vi "main.vi"() -> (0 "error out":errorcluster)   [LabVIEW 2012]
uses:
  Global1.vi
  <vilib>/Utility/file.llb/Read From Spreadsheet File (string).vi
panel:
  out "element":string
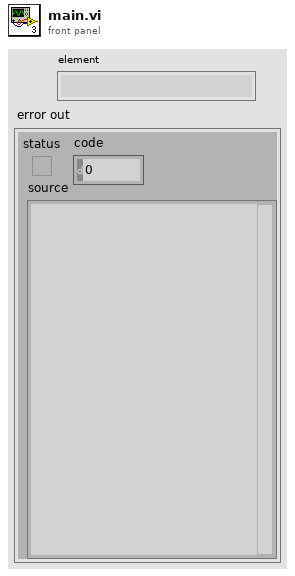
[diagram p1: front panel]
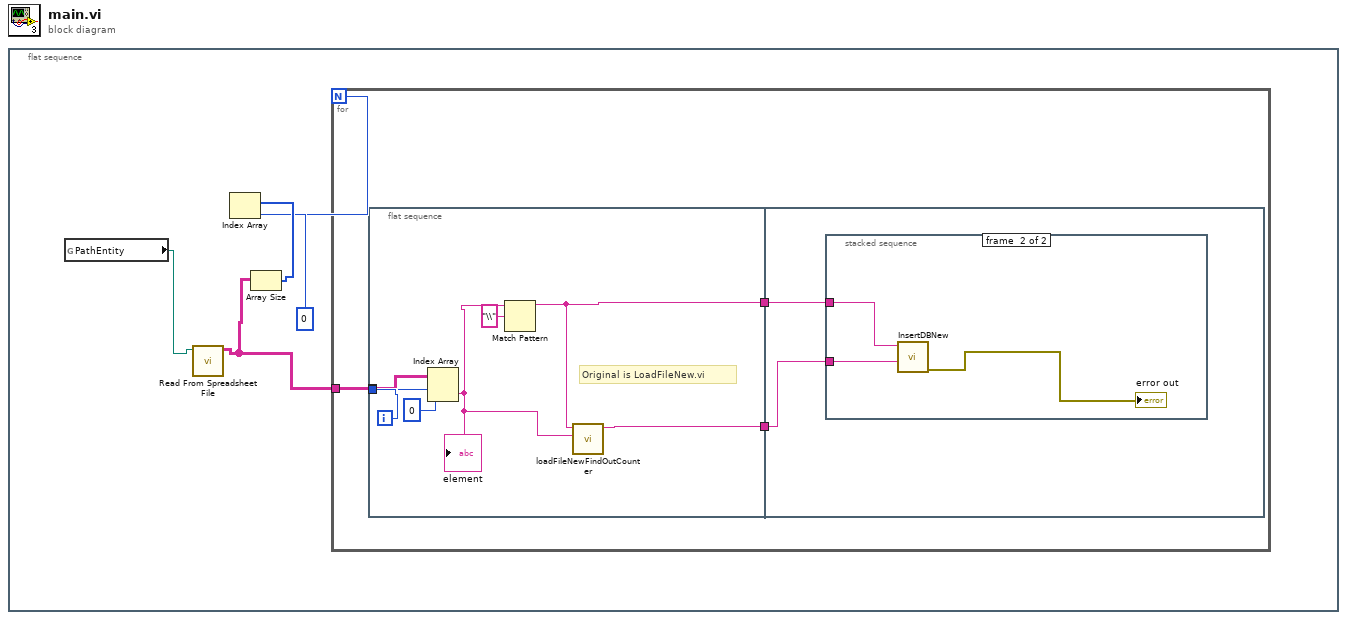
[diagram p0: block diagram]
diagram:
  n1 = flat-sequence {
    frame #0 {
      n2 = global read "Global1.vi" "PathEntity"() -> (w1:path)
      n3 = call-poly <vilib>:"Read From Spreadsheet File.vi"("file path (dialog if empty)"=w1) -> ("all rows"=w2:string[][])  [unwired: 6 in, 4 out]
      n4 = Array Size(array=w2) -> (size(s)=w5:i32[])
      n5 = Index Array(array=w5, index=0) -> (element=w3:i32)
      n6 = for {
        N: w3 -> [_]
        tunnel: w2 -> [w9]
        i -> [w8]
        n7 = flat-sequence {
          tunnel: w9 -> [w16]
          tunnel: w8 -> [w14]
          tunnel: [w11] -> w7
          tunnel: [w10] -> w6
          tunnel: w7 -> [w18]
          tunnel: w6 -> [w17]
          frame #0 {
            # "Original is LoadFileNew.vi"
            n8 = Index Array(array=w16, index (row)=w14, index (col)=0 ("disabled index (col)")) -> (element=w12:string)
            "element" <- w12
            n9 = Match Pattern(string=w12, regular expression="\\") -> (before substring=w10:string)  [unwired: 1 in, 3 out]
            n10 = call "loadFileNewFindOutCounter.vi"("folder"=w12, "Entity"=w10) -> ("Lot"=w11:string)  [unwired: 8 in, 1 out]
          }
          frame #1 {
            n11 = stacked-sequence {
              tunnel: w18 -> [_ w21]
              tunnel: w17 -> [_ w20]
              frame #0 {
                # "html2dbnew.vi"
              }
              frame #1 {
                n12 = call "InsertDBNew.vi"("String"=w21, "Entity"=w20) -> ("error out"=→"error out":errorcluster)  [unwired: 9 in]
              }
            }
          }
        }
      }
    }
  }
